vi "set_NP_Select.vi"(0 "N/P Dopant DA Switch":bool) -> ()   [LabVIEW 2011]
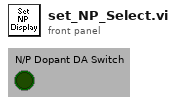
[diagram p1: front panel]
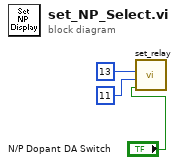
[diagram p0: block diagram]
diagram:
  n1 = call "set_relay.vi"("Slot"=13, "Relay"=11, "Relay Status"="N/P Dopant DA Switch") -> ()  [unwired: 1 in, 2 out]
